vi "vision board.vi"(8 "error in (no error)":errorcluster) -> (0 "error out":errorcluster, 2 "vision board":T1, 3 "recycle?":bool)   [LabVIEW 2019]
uses:
  vision/vision_board_ctl.ctl
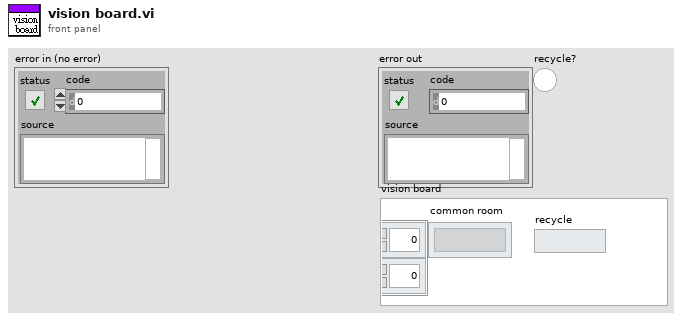
[diagram p1: front panel]
types:
  T1 = typedef "vision_board_ctl.ctl" = cluster{"common room":string[][], "recycle":string}
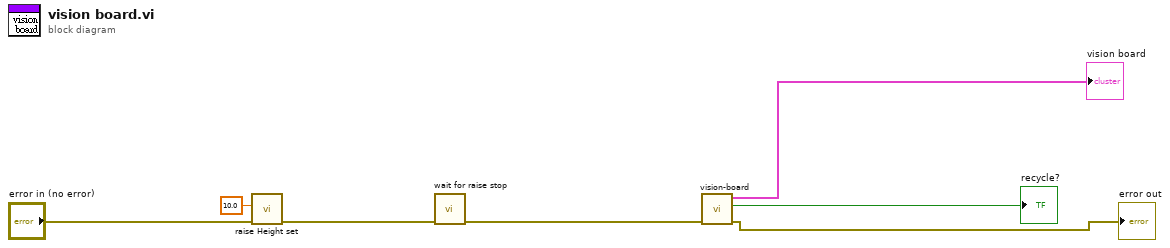
[diagram p0: block diagram]
diagram:
  n1 = call "raise Height set.vi"("error in (no error)"="error in (no error)", "Height_cm"=10.0) -> ("error out"=w2:errorcluster)  [unwired: 9 in]
  n2 = call "wait for raise stop.vi"("Error In"=w2) -> ("Error Out"=w1:errorcluster)  [unwired: 10 in]
  n3 = call "vision-board.vi"("error in"=w1) -> ("error out"=→"error out":errorcluster, "recycle?"=→"recycle?":bool, "vision board"=→"vision board":T1)  [unwired: 8 in]
